vi "auto cross defense.vi"(8 "Defense type":dbl, 11 "Distance":dbl=24.0 format="%#_13g") -> ()   [LabVIEW 2015]
uses:
  <vilib>/Rock Robotics/WPI/Solenoid/WPI_SolenoidValue.ctl
  <vilib>/Rock Robotics/WPI/Solenoid/WPI_SolenoidSetEnum.vi
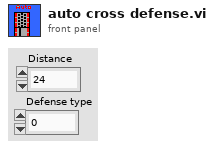
[diagram p1: front panel]
types:
  T1 = typedef "WPI_MotorControlDeviceRef.ctl" = cluster{"DeviceStatus":errorcluster, "Type":T2, "PWM":cluster{"PWM Channel":T3, "DeadBand":T4}, "CAN":cluster{"Device Number":u8, "Control Mode":T5, "Semaphore":T6, "Max Vout":dbl, "TalonSRX Control Mode":T7}, "Invert":bool}
  T2 = typedef "WPI_MotorControlType.ctl" = enum16{"PWM", "CAN", "CANTalonSRX"}
  T3 = typedef "FPGA_DIOPWMChannel.ctl" = enum8{"PWM 0", "PWM 1", "PWM 2", "PWM 3", "PWM 4", "PWM 5", "PWM 6", "PWM 7", "PWM 8", "PWM 9", "PWM MXP 0", "PWM MXP 1", "PWM MXP 2", "PWM MXP 3", "PWM MXP 4", "PWM MXP 5", "PWM MXP 6", "PWM MXP 7", "PWM MXP 8", "PWM MXP 9", "Invalid"}
  T4 = typedef "WPI_PWMDeadband.ctl" = cluster{"Name":string, "maxPositivePwm":i32, "minPositivePwm":i32, "centerPwm":i32, "maxNegativePwm":i32, "minNegativePwm":i32, "angularRange":u16}
  T5 = typedef "WPI_CANJaguar_ControlMode.ctl" = enum8{"Percent VBus", "Current", "Speed", "Position", "Voltage"}
  T6 = typedef "Semaphore RefNum" = refnum<k1>
  T7 = typedef "WPI_CANTalonSRX_APIControlMode.ctl" = enum8{"Percent VBus", "Speed", "Position", "Slave", "Unchanged / Invalid", "Voltage Compensation", "Current", "Motion Profile"}
  T8 = typedef "WPI_SolenoidDevRef.ctl" = cluster{"DevStatus":errorcluster, "Pneumatics Control Module":u8, "Forward Solenoid Channel":T9, "Reverse Solenoid Channel":T9}
  T9 = typedef "WPI_SolenoidChannel.ctl" = enum8{"Solenoid 0", "Solenoid 1", "Solenoid 2", "Solenoid 3", "Solenoid 4", "Solenoid 5", "Solenoid 6", "Solenoid 7", "Invalid"}
  T10 = typedef "WPI_SolenoidValue.ctl" = enum16{"Off", "On", "Forward", "Reverse"}
  T11 = typedef "WPI_CANTalonSRX_GlobalStatus.ctl" = cluster{"Applied Throttle":dbl, "Module Enabled":bool, "CAN Error":errorcluster, "Closed Loop Error":dbl, "Forward Limit Switch Closed":bool, "Reverse Limit Switch Closed":bool, "Sensor Position":dbl, "Sensor Velocity":dbl, "Current":dbl, "Sticky Fault - Over Temp":bool, "Sticky Fault - Under Voltage":bool, "Sticky Fault - Forward Limit":bool, "Sticky Fault - Reverse Limit":bool, "Sticky Fault - Forward Soft Limit":bool, "Sticky Fault - Reverse Soft Limit":bool, "Brake is Enabled":bool, "Encoder Position":dbl, "Encoder Velocity":dbl, "Encoder Index Count":dbl, "Encoder A Pin State":bool, "Encoder B Pin State":bool, "Encoder Index Pin State":bool, "Analog In":dbl, "Analog In Velocity":dbl, "Temperature (C)":dbl, "Battery Voltage":dbl, "Control 5 Is Supported":bool, "Current Profile Slot Select":dbl, "Pos Div 8":bool, "Vel Div 4":bool, "Pulse Width Position":i32, "Pulse Width Velocity":i32, "Pulse Width Rise To Rise (us)":i32, "Pulse Width Rise To Fall (us)":i32, "Mot Prof Active Is Under Run":bool, "Mot Prof Active Has Under Run":bool, "Mot Prof Active Is Last":bool, "Mot Prof Active Velocity Only":bool, "Mot Prof Active Is Valid":bool, "Mot Prof Buffer Is Full":bool, "Mot Prof Active Profile Slot Select":i32, "Mot Prof NextID":i32, "Mot Prof Count":i32, "Mot Prof Active Velocity":dbl, "Mot Prof Active Position":dbl, "Mot Prof Output Enable":i32}
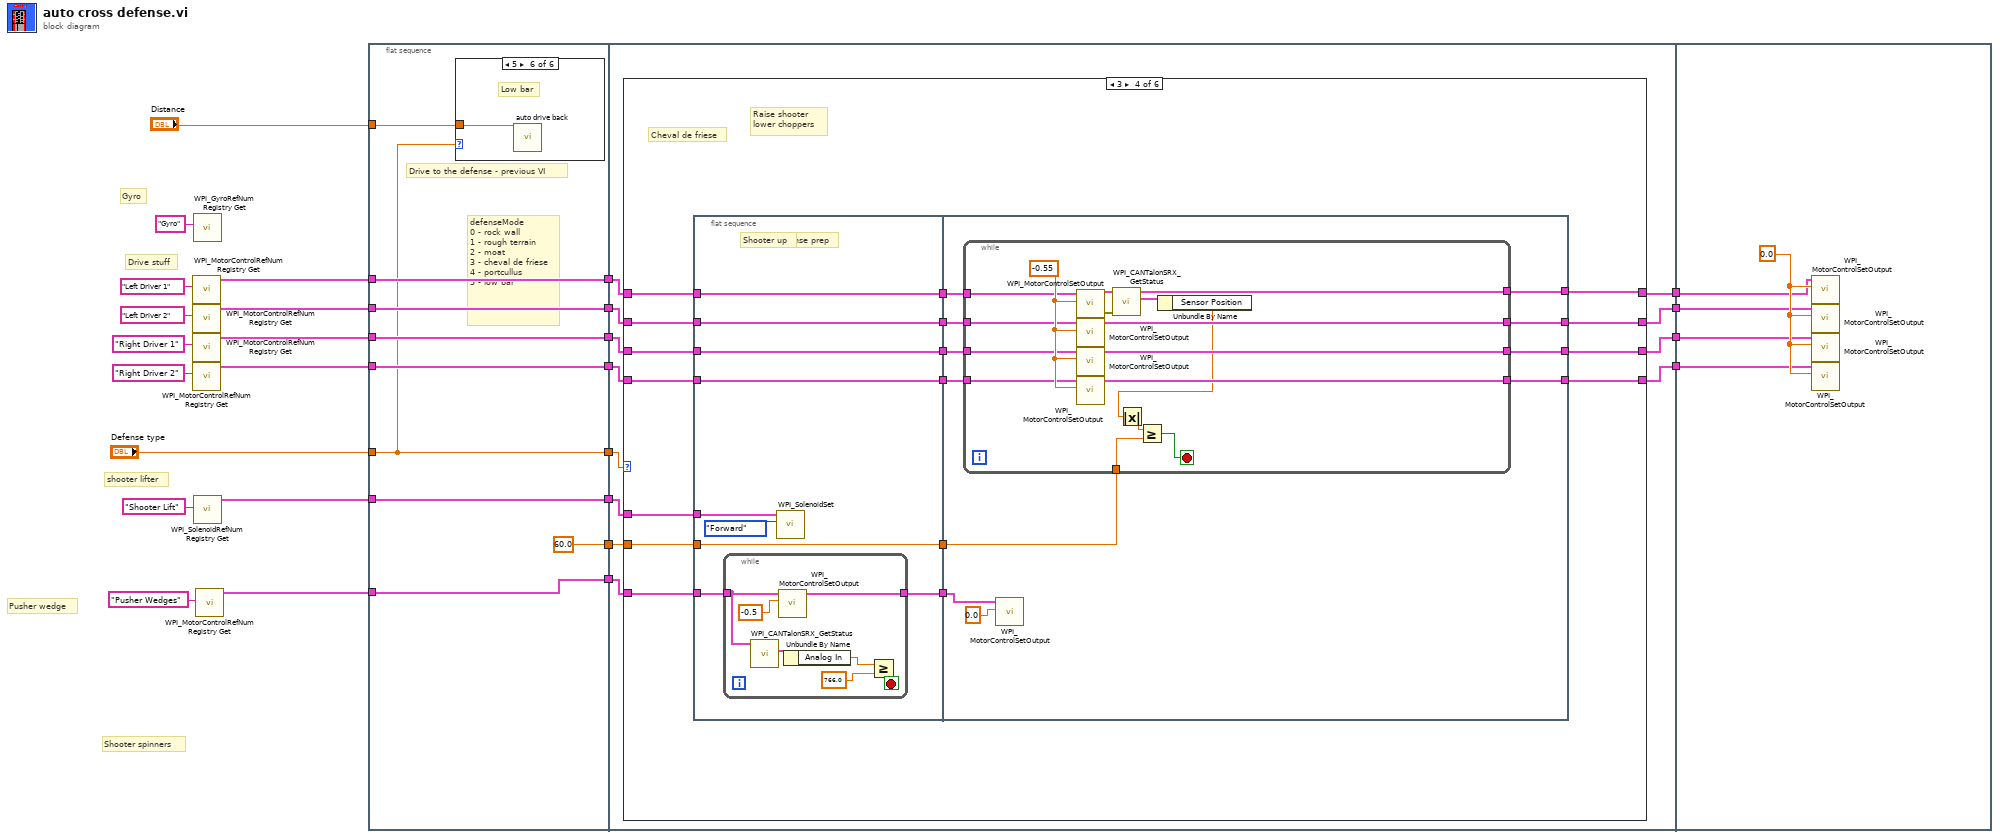
[diagram p0: block diagram]
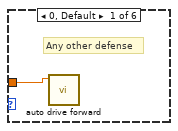
[diagram p2: hidden frame]
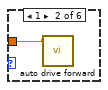
[diagram p3: hidden frame]
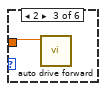
[diagram p4: hidden frame]
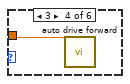
[diagram p5: hidden frame]
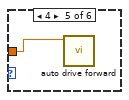
[diagram p6: hidden frame]
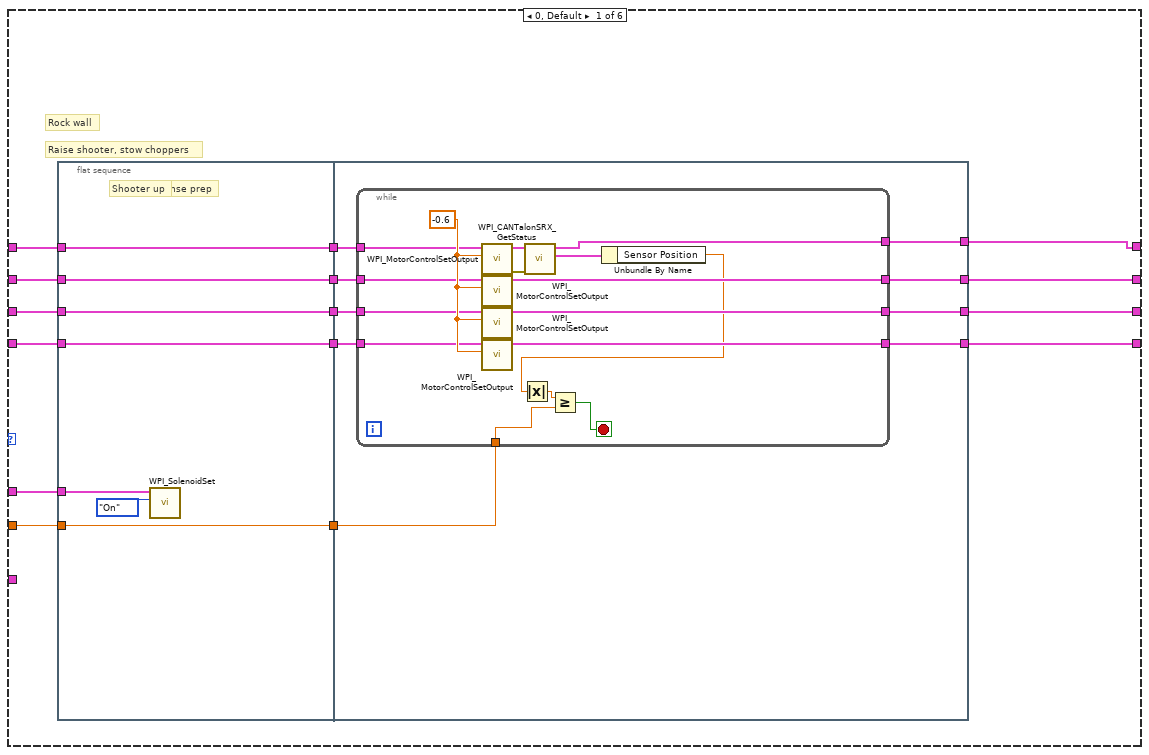
[diagram p7: hidden frame]
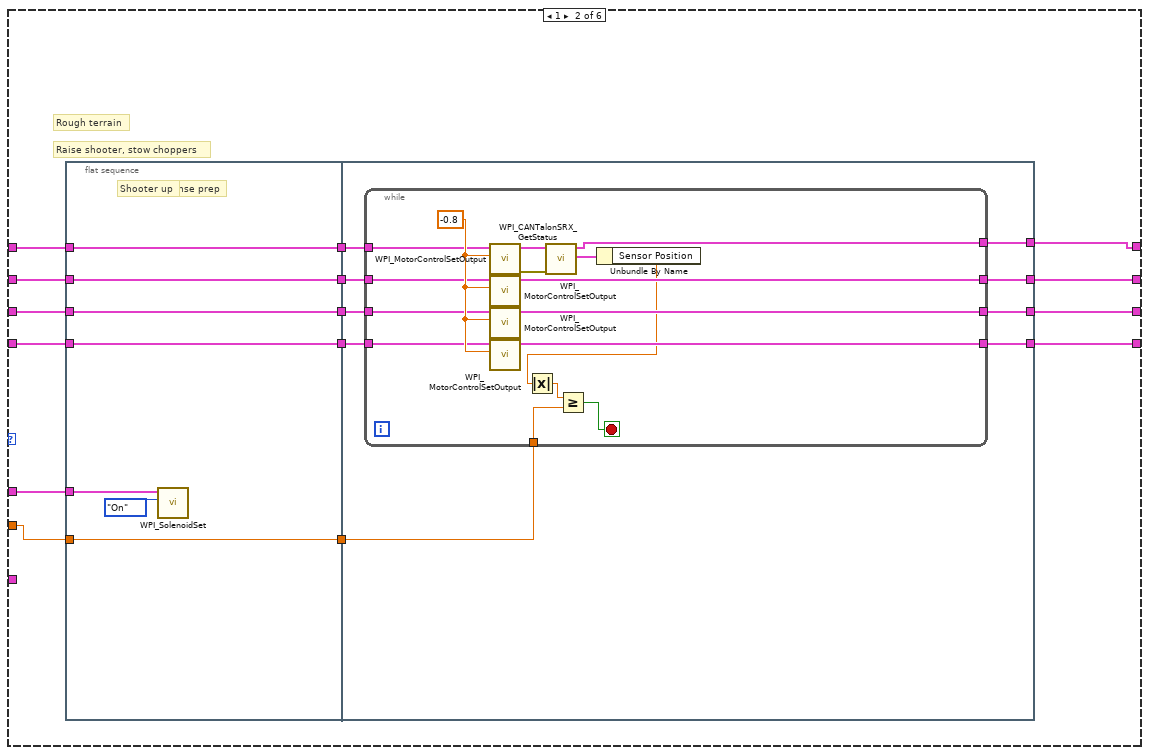
[diagram p8: hidden frame]
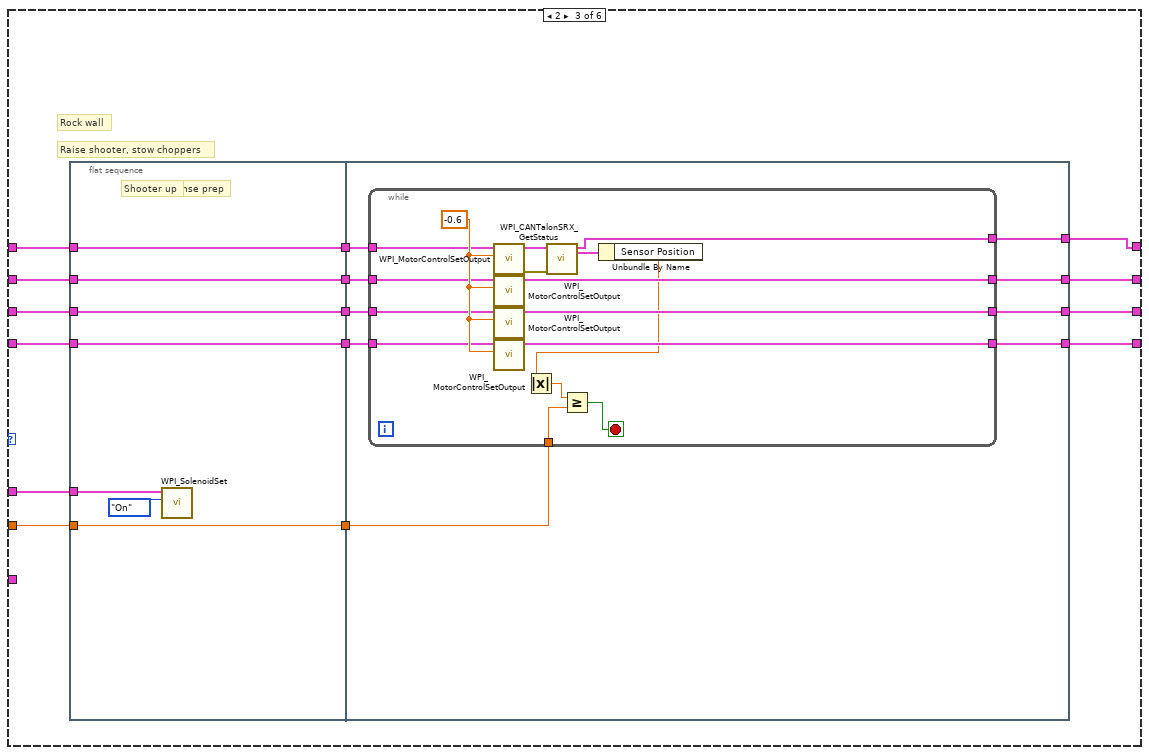
[diagram p9: hidden frame]
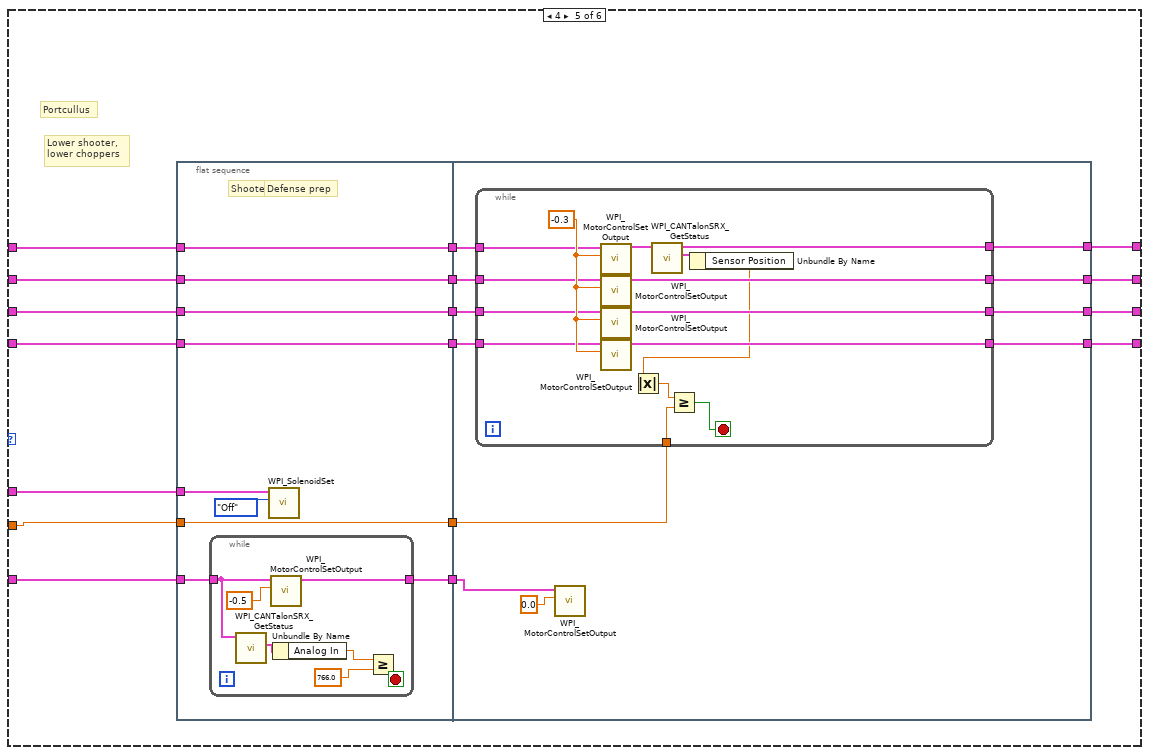
[diagram p10: hidden frame]
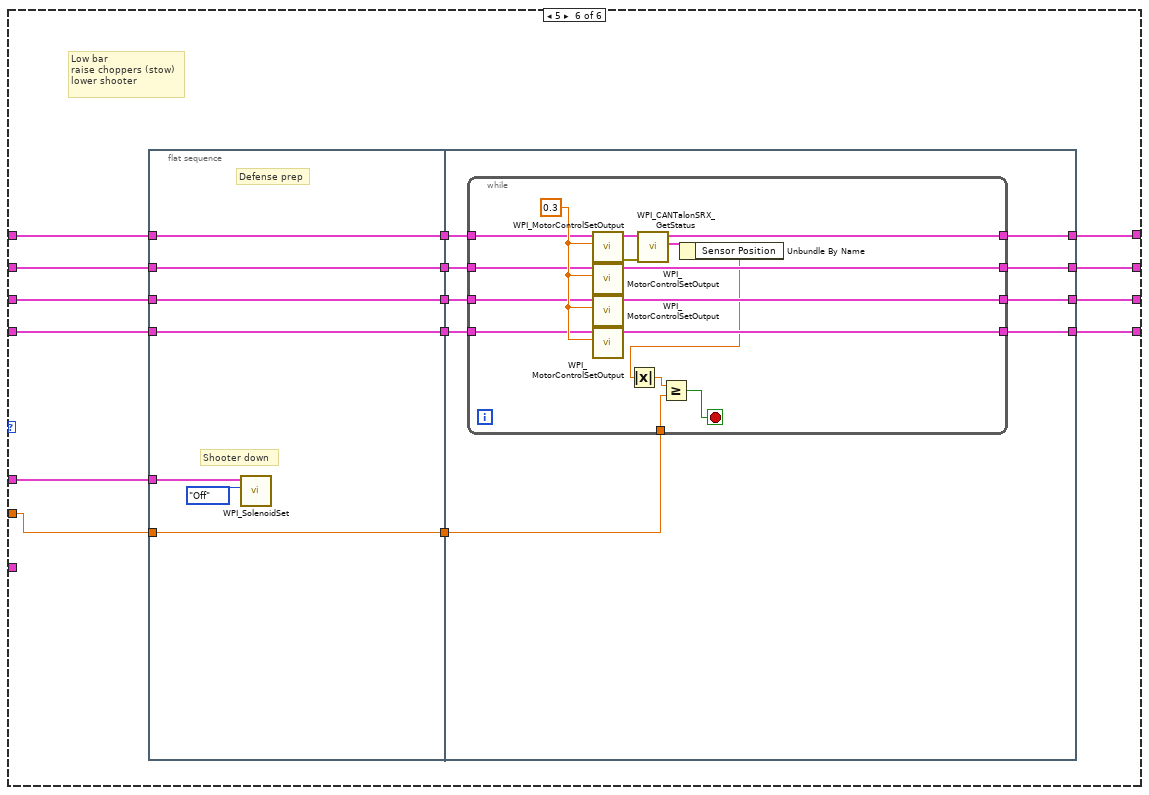
[diagram p11: hidden frame]
diagram:
  # "Pusher wedge"
  # "Shooter spinners"
  # "shooter lifter"
  # "Drive stuff"
  # "Gyro"
  n1 = call <vilib>:"WPI_MotorControlRefNum Registry Get.vi"("refnum name"="Left Driver 1") -> ("MotorControlDevRef"=w17:T1)  [unwired: 9 in, 1 out]
  n2 = call <vilib>:"WPI_MotorControlRefNum Registry Get.vi"("refnum name"="Left Driver 2") -> ("MotorControlDevRef"=w15:T1)  [unwired: 9 in, 1 out]
  n3 = call <vilib>:"WPI_MotorControlRefNum Registry Get.vi"("refnum name"="Right Driver 1") -> ("MotorControlDevRef"=w14:T1)  [unwired: 9 in, 1 out]
  n4 = call <vilib>:"WPI_MotorControlRefNum Registry Get.vi"("refnum name"="Right Driver 2") -> ("MotorControlDevRef"=w11:T1)  [unwired: 9 in, 1 out]
  n5 = call <vilib>:"WPI_GyroRefNum Registry Get.vi"("refnum name"="Gyro") -> ()  [unwired: 9 in, 2 out]
  n6 = call <vilib>:"WPI_SolenoidRefNum Registry Get.vi"("refnum name"="Shooter Lift") -> ("SolenoidDevRef"=w20:T8)  [unwired: 9 in, 1 out]
  n7 = call <vilib>:"WPI_MotorControlRefNum Registry Get.vi"("refnum name"="Pusher Wedges") -> ("MotorControlDevRef"=w3:T1)  [unwired: 9 in, 1 out]
  n8 = flat-sequence {
    tunnel: [w30] -> w21
    tunnel: "Defense type" -> [w30]
    tunnel: w20 -> [w36]
    tunnel: [w36] -> w19
    tunnel: [w35] -> w18
    tunnel: w17 -> [w35]
    tunnel: [w34] -> w16
    tunnel: w15 -> [w34]
    tunnel: w14 -> [w33]
    tunnel: [w33] -> w13
    tunnel: [w32] -> w12
    tunnel: w11 -> [w32]
    tunnel: "Distance" -> [w31]
    tunnel: [w29] -> w4
    tunnel: w3 -> [w29]
    tunnel: [60.0 ("y")] -> w2
    tunnel: w21 -> [w54]
    tunnel: w19 -> [w53]
    tunnel: w18 -> [w52]
    tunnel: w16 -> [w51]
    tunnel: w13 -> [w50]
    tunnel: w12 -> [w49]
    tunnel: [w48] -> w10
    tunnel: [w47] -> w9
    tunnel: [w46] -> w8
    tunnel: w4 -> [w45]
    tunnel: w2 -> [w44]
    tunnel: [w43] -> w1
    tunnel: w10 -> [w365]
    tunnel: w9 -> [w364]
    tunnel: w8 -> [w363]
    tunnel: w1 -> [w362]
    frame #0 {
      # "defenseMode\n0 - rock wall\n1 - rough terrain\n2 - moat\n3 - cheval de friese\n4 - portcullus\n5 - low bar"
      # "Drive to the defense - previous VI"
      n9 = case shown="5" w30 {
        tunnel: w31 -> [w37 w38 w39 w40 w41 w42]
        frame 0, Default {
          # "Any other defense"
          n10 = call "auto drive forward.vi"("Distance"=w37) -> ()  [unwired: 11 in]
        }
        frame 1 {
          n11 = call "auto drive forward.vi"("Distance"=w38) -> ()  [unwired: 11 in]
        }
        frame 2 {
          n12 = call "auto drive forward.vi"("Distance"=w39) -> ()  [unwired: 11 in]
        }
        frame 3 {
          n13 = call "auto drive forward.vi"("Distance"=w40) -> ()  [unwired: 11 in]
        }
        frame 4 {
          n14 = call "auto drive forward.vi"("Distance"=w41) -> ()  [unwired: 11 in]
        }
        frame 5 {
          # "Low bar"
          n15 = call "auto drive back.vi"("Distance"=w42) -> ()  [unwired: 11 in]
        }
      }
    }
    frame #1 {
      n16 = case shown="3" w54 {
        tunnel: w53 -> [w69 w108 w155 w203 w264 w321]
        tunnel: w52 -> [w67 w112 w159 w207 w268 w325]
        tunnel: w51 -> [w65 w111 w158 w206 w267 w324]
        tunnel: w50 -> [w64 w110 w157 w205 w266 w323]
        tunnel: w49 -> [w61 w109 w156 w204 w265 w322]
        tunnel: [w60 w107 w154 w202 w262 w318] -> w48
        tunnel: [w59 w106 w153 w201 w261 w319] -> w47
        tunnel: [w58 w105 w152 w200 w260 w320] -> w46
        tunnel: w45 -> [_ _ _ w199 w259 _]
        tunnel: w44 -> [w57 w104 w150 w198 w258 w317]
        tunnel: [w55 w102 w149 w196 w256 w315] -> w43
        frame 0, Default {
          # "Raise shooter, stow choppers"
          # "Rock wall"
          n17 = flat-sequence {
            tunnel: w69 -> [w76]
            tunnel: [w74] -> w68
            tunnel: w67 -> [w74]
            tunnel: [w73] -> w66
            tunnel: w65 -> [w73]
            tunnel: w64 -> [w72]
            tunnel: [w72] -> w63
            tunnel: [w71] -> w62
            tunnel: w61 -> [w71]
            tunnel: w57 -> [w70]
            tunnel: [w70] -> w56
            tunnel: w68 -> [w85]
            tunnel: w66 -> [w84]
            tunnel: w63 -> [w83]
            tunnel: w62 -> [w82]
            tunnel: [w81] -> w60
            tunnel: [w80] -> w59
            tunnel: [w79] -> w58
            tunnel: w56 -> [w78]
            tunnel: [w77] -> w55
            frame #0 {
              # "Defense prep"
              # "Shooter up"
              n18 = call-poly <vilib>:"WPI_SolenoidSet.vi"("Value"=WPI_SolenoidValue."On", "SolenoidDevRef"=w76) -> ()  [unwired: 8 in, 2 out]
            }
            frame #1 {
              n19 = while {
                tunnel: w85 -> [w100]
                tunnel: w84 -> [w99]
                tunnel: w83 -> [w98]
                tunnel: w82 -> [w97]
                tunnel: [w95] -> w81
                tunnel: [w94] -> w80
                tunnel: [w93] -> w79
                tunnel: w78 -> [w92]
                tunnel: [w86] -> w77
                stop <- w96 stop-if-true
                w101 = -0.6
                n20 = call <vilib>:"WPI_MotorControlSetOutput.vi"("Output"=w101, "MotorControlDevRef"=w100) -> ("error out"=w91:errorcluster, "MotorControlDevRef"=w90:T1)  [unwired: 7 in, 1 out]
                n21 = call <vilib>:"WPI_MotorControlSetOutput.vi"("Output"=w101, "MotorControlDevRef"=w99) -> ("MotorControlDevRef"=w95:T1)  [unwired: 7 in, 2 out]
                n22 = call <vilib>:"WPI_MotorControlSetOutput.vi"("Output"=w101, "MotorControlDevRef"=w98) -> ("MotorControlDevRef"=w94:T1)  [unwired: 7 in, 2 out]
                n23 = call <vilib>:"WPI_MotorControlSetOutput.vi"("Output"=w101, "MotorControlDevRef"=w97) -> ("MotorControlDevRef"=w93:T1)  [unwired: 7 in, 2 out]
                n24 = call <vilib>:"WPI_CANTalonSRX_GetStatus.vi"("error in (no error)"=w91, "CAN Talon SRX Ref"=w90) -> ("Talon SRX Status"=w89:T11, "CAN Talon SRX Ref"=w86:T1)  [unwired: 7 in, 1 out]
                n25 = Unbundle By Name(w89) -> ("Sensor Position"=w87:dbl)
                n26 = Absolute Value(x=w87) -> (abs(x)=w88:dbl)
                n27 = Greater Or Equal?(x=w88, y=w92) -> (x >= y?=w96:bool)
              }
            }
          }
        }
        frame 1 {
          # "Raise shooter, stow choppers"
          # "Rough terrain"
          n28 = flat-sequence {
            tunnel: w108 -> [w123]
            tunnel: [w121] -> w116
            tunnel: w112 -> [w121]
            tunnel: [w120] -> w115
            tunnel: w111 -> [w120]
            tunnel: w110 -> [w119]
            tunnel: [w119] -> w114
            tunnel: [w118] -> w113
            tunnel: w109 -> [w118]
            tunnel: w104 -> [w117]
            tunnel: [w117] -> w103
            tunnel: w116 -> [w132]
            tunnel: w115 -> [w131]
            tunnel: w114 -> [w130]
            tunnel: w113 -> [w129]
            tunnel: [w128] -> w107
            tunnel: [w127] -> w106
            tunnel: [w126] -> w105
            tunnel: w103 -> [w125]
            tunnel: [w124] -> w102
            frame #0 {
              # "Defense prep"
              # "Shooter up"
              n29 = call-poly <vilib>:"WPI_SolenoidSet.vi"("Value"=WPI_SolenoidValue."On", "SolenoidDevRef"=w123) -> ()  [unwired: 8 in, 2 out]
            }
            frame #1 {
              n30 = while {
                tunnel: w132 -> [w147]
                tunnel: w131 -> [w146]
                tunnel: w130 -> [w145]
                tunnel: w129 -> [w144]
                tunnel: [w142] -> w128
                tunnel: [w141] -> w127
                tunnel: [w140] -> w126
                tunnel: w125 -> [w138]
                tunnel: [w133] -> w124
                stop <- w143 stop-if-true
                w148 = -0.8
                n31 = call <vilib>:"WPI_MotorControlSetOutput.vi"("Output"=w148, "MotorControlDevRef"=w147) -> ("error out"=w137:errorcluster, "MotorControlDevRef"=w136:T1)  [unwired: 7 in, 1 out]
                n32 = call <vilib>:"WPI_MotorControlSetOutput.vi"("Output"=w148, "MotorControlDevRef"=w146) -> ("MotorControlDevRef"=w142:T1)  [unwired: 7 in, 2 out]
                n33 = call <vilib>:"WPI_MotorControlSetOutput.vi"("Output"=w148, "MotorControlDevRef"=w145) -> ("MotorControlDevRef"=w141:T1)  [unwired: 7 in, 2 out]
                n34 = call <vilib>:"WPI_MotorControlSetOutput.vi"("Output"=w148, "MotorControlDevRef"=w144) -> ("MotorControlDevRef"=w140:T1)  [unwired: 7 in, 2 out]
                n35 = call <vilib>:"WPI_CANTalonSRX_GetStatus.vi"("error in (no error)"=w137, "CAN Talon SRX Ref"=w136) -> ("Talon SRX Status"=w135:T11, "CAN Talon SRX Ref"=w133:T1)  [unwired: 7 in, 1 out]
                n36 = Unbundle By Name(w135) -> ("Sensor Position"=w134:dbl)
                n37 = Absolute Value(x=w134) -> (abs(x)=w139:dbl)
                n38 = Greater Or Equal?(x=w139, y=w138) -> (x >= y?=w143:bool)
              }
            }
          }
        }
        frame 2 {
          # "Raise shooter, stow choppers"
          # "Rock wall"
          n39 = flat-sequence {
            tunnel: w155 -> [w170]
            tunnel: [w168] -> w163
            tunnel: w159 -> [w168]
            tunnel: [w167] -> w162
            tunnel: w158 -> [w167]
            tunnel: w157 -> [w166]
            tunnel: [w166] -> w161
            tunnel: [w165] -> w160
            tunnel: w156 -> [w165]
            tunnel: [w164] -> w151
            tunnel: w150 -> [w164]
            tunnel: w163 -> [w179]
            tunnel: w162 -> [w178]
            tunnel: w161 -> [w177]
            tunnel: w160 -> [w176]
            tunnel: [w175] -> w154
            tunnel: [w174] -> w153
            tunnel: [w173] -> w152
            tunnel: w151 -> [w172]
            tunnel: [w171] -> w149
            frame #0 {
              # "Defense prep"
              # "Shooter up"
              n40 = call-poly <vilib>:"WPI_SolenoidSet.vi"("Value"=WPI_SolenoidValue."On", "SolenoidDevRef"=w170) -> ()  [unwired: 8 in, 2 out]
            }
            frame #1 {
              n41 = while {
                tunnel: w179 -> [w194]
                tunnel: w178 -> [w193]
                tunnel: w177 -> [w192]
                tunnel: w176 -> [w191]
                tunnel: [w189] -> w175
                tunnel: [w188] -> w174
                tunnel: [w187] -> w173
                tunnel: w172 -> [w185]
                tunnel: [w180] -> w171
                stop <- w190 stop-if-true
                w195 = -0.6
                n42 = call <vilib>:"WPI_MotorControlSetOutput.vi"("Output"=w195, "MotorControlDevRef"=w194) -> ("error out"=w184:errorcluster, "MotorControlDevRef"=w183:T1)  [unwired: 7 in, 1 out]
                n43 = call <vilib>:"WPI_MotorControlSetOutput.vi"("Output"=w195, "MotorControlDevRef"=w193) -> ("MotorControlDevRef"=w189:T1)  [unwired: 7 in, 2 out]
                n44 = call <vilib>:"WPI_MotorControlSetOutput.vi"("Output"=w195, "MotorControlDevRef"=w192) -> ("MotorControlDevRef"=w188:T1)  [unwired: 7 in, 2 out]
                n45 = call <vilib>:"WPI_MotorControlSetOutput.vi"("Output"=w195, "MotorControlDevRef"=w191) -> ("MotorControlDevRef"=w187:T1)  [unwired: 7 in, 2 out]
                n46 = call <vilib>:"WPI_CANTalonSRX_GetStatus.vi"("error in (no error)"=w184, "CAN Talon SRX Ref"=w183) -> ("Talon SRX Status"=w182:T11, "CAN Talon SRX Ref"=w180:T1)  [unwired: 7 in, 1 out]
                n47 = Unbundle By Name(w182) -> ("Sensor Position"=w181:dbl)
                n48 = Absolute Value(x=w181) -> (abs(x)=w186:dbl)
                n49 = Greater Or Equal?(x=w186, y=w185) -> (x >= y?=w190:bool)
              }
            }
          }
        }
        frame 3 {
          # "Raise shooter\nlower choppers"
          # "Cheval de friese"
          n50 = flat-sequence {
            tunnel: w203 -> [w221]
            tunnel: [w219] -> w212
            tunnel: w207 -> [w219]
            tunnel: [w218] -> w211
            tunnel: w206 -> [w218]
            tunnel: w205 -> [w217]
            tunnel: [w217] -> w210
            tunnel: [w216] -> w209
            tunnel: w204 -> [w216]
            tunnel: [w215] -> w208
            tunnel: w199 -> [w214]
            tunnel: w198 -> [w213]
            tunnel: [w213] -> w197
            tunnel: w212 -> [w239]
            tunnel: w211 -> [w238]
            tunnel: w210 -> [w237]
            tunnel: w209 -> [w236]
            tunnel: w208 -> [w231]
            tunnel: w197 -> [w230]
            tunnel: [w235] -> w202
            tunnel: [w234] -> w201
            tunnel: [w233] -> w200
            tunnel: [w229] -> w196
            frame #0 {
              # "Defense prep"
              # "Shooter up"
              n51 = while {
                tunnel: [w227] -> w215
                tunnel: w214 -> [w222]
                stop <- w223 stop-if-true
                n52 = call <vilib>:"WPI_CANTalonSRX_GetStatus.vi"("CAN Talon SRX Ref"=w222) -> ("Talon SRX Status"=w225:T11)  [unwired: 8 in, 2 out]
                n53 = call <vilib>:"WPI_MotorControlSetOutput.vi"("Output"=-0.5, "MotorControlDevRef"=w222) -> ("MotorControlDevRef"=w227:T1)  [unwired: 7 in, 2 out]
                n54 = Unbundle By Name(w225) -> ("Analog In"=w224:dbl)
                n55 = Greater Or Equal?(x=w224, y=766.0) -> (x >= y?=w223:bool)
              }
              n56 = call-poly <vilib>:"WPI_SolenoidSet.vi"("Value"=WPI_SolenoidValue."Forward", "SolenoidDevRef"=w221) -> ()  [unwired: 8 in, 2 out]
            }
            frame #1 {
              n57 = while {
                tunnel: w239 -> [w254]
                tunnel: w238 -> [w253]
                tunnel: w237 -> [w252]
                tunnel: w236 -> [w251]
                tunnel: [w249] -> w235
                tunnel: [w248] -> w234
                tunnel: [w247] -> w233
                tunnel: w230 -> [w245]
                tunnel: [w240] -> w229
                stop <- w250 stop-if-true
                w255 = -0.55
                n58 = call <vilib>:"WPI_MotorControlSetOutput.vi"("Output"=w255, "MotorControlDevRef"=w254) -> ("error out"=w243:errorcluster, "MotorControlDevRef"=w244:T1)  [unwired: 7 in, 1 out]
                n59 = call <vilib>:"WPI_MotorControlSetOutput.vi"("Output"=w255, "MotorControlDevRef"=w253) -> ("MotorControlDevRef"=w249:T1)  [unwired: 7 in, 2 out]
                n60 = call <vilib>:"WPI_MotorControlSetOutput.vi"("Output"=w255, "MotorControlDevRef"=w252) -> ("MotorControlDevRef"=w248:T1)  [unwired: 7 in, 2 out]
                n61 = call <vilib>:"WPI_MotorControlSetOutput.vi"("Output"=w255, "MotorControlDevRef"=w251) -> ("MotorControlDevRef"=w247:T1)  [unwired: 7 in, 2 out]
                n62 = call <vilib>:"WPI_CANTalonSRX_GetStatus.vi"("error in (no error)"=w243, "CAN Talon SRX Ref"=w244) -> ("Talon SRX Status"=w242:T11, "CAN Talon SRX Ref"=w240:T1)  [unwired: 7 in, 1 out]
                n63 = Unbundle By Name(w242) -> ("Sensor Position"=w241:dbl)
                n64 = Absolute Value(x=w241) -> (abs(x)=w246:dbl)
                n65 = Greater Or Equal?(x=w246, y=w245) -> (x >= y?=w250:bool)
              }
              n66 = call <vilib>:"WPI_MotorControlSetOutput.vi"("Output"=0.0, "MotorControlDevRef"=w231) -> ()  [unwired: 7 in, 3 out]
            }
          }
        }
        frame 4 {
          # "Lower shooter,\nlower choppers"
          # "Portcullus"
          n67 = flat-sequence {
            tunnel: w264 -> [w281]
            tunnel: [w279] -> w272
            tunnel: w268 -> [w279]
            tunnel: [w278] -> w271
            tunnel: w267 -> [w278]
            tunnel: w266 -> [w277]
            tunnel: [w277] -> w270
            tunnel: [w276] -> w269
            tunnel: w265 -> [w276]
            tunnel: [w275] -> w263
            tunnel: w259 -> [w274]
            tunnel: w258 -> [w273]
            tunnel: [w273] -> w257
            tunnel: w272 -> [w299]
            tunnel: w271 -> [w298]
            tunnel: w270 -> [w297]
            tunnel: w269 -> [w296]
            tunnel: w263 -> [w291]
            tunnel: w257 -> [w290]
            tunnel: [w295] -> w262
            tunnel: [w294] -> w261
            tunnel: [w293] -> w260
            tunnel: [w289] -> w256
            frame #0 {
              # "Defense prep"
              # "Shooter down"
              n68 = while {
                tunnel: [w287] -> w275
                tunnel: w274 -> [w282]
                stop <- w283 stop-if-true
                n69 = call <vilib>:"WPI_CANTalonSRX_GetStatus.vi"("CAN Talon SRX Ref"=w282) -> ("Talon SRX Status"=w285:T11)  [unwired: 8 in, 2 out]
                n70 = call <vilib>:"WPI_MotorControlSetOutput.vi"("Output"=-0.5, "MotorControlDevRef"=w282) -> ("MotorControlDevRef"=w287:T1)  [unwired: 7 in, 2 out]
                n71 = Unbundle By Name(w285) -> ("Analog In"=w284:dbl)
                n72 = Greater Or Equal?(x=w284, y=766.0) -> (x >= y?=w283:bool)
              }
              n73 = call-poly <vilib>:"WPI_SolenoidSet.vi"("Value"=WPI_SolenoidValue."Off", "SolenoidDevRef"=w281) -> ()  [unwired: 8 in, 2 out]
            }
            frame #1 {
              n74 = while {
                tunnel: w299 -> [w313]
                tunnel: w298 -> [w312]
                tunnel: w297 -> [w311]
                tunnel: w296 -> [w310]
                tunnel: [w308] -> w295
                tunnel: [w307] -> w294
                tunnel: [w306] -> w293
                tunnel: w290 -> [w304]
                tunnel: [w302] -> w289
                stop <- w309 stop-if-true
                w314 = -0.3
                n75 = call <vilib>:"WPI_MotorControlSetOutput.vi"("Output"=w314, "MotorControlDevRef"=w313) -> ("MotorControlDevRef"=w303:T1)  [unwired: 7 in, 2 out]
                n76 = call <vilib>:"WPI_MotorControlSetOutput.vi"("Output"=w314, "MotorControlDevRef"=w312) -> ("MotorControlDevRef"=w308:T1)  [unwired: 7 in, 2 out]
                n77 = call <vilib>:"WPI_MotorControlSetOutput.vi"("Output"=w314, "MotorControlDevRef"=w311) -> ("MotorControlDevRef"=w307:T1)  [unwired: 7 in, 2 out]
                n78 = call <vilib>:"WPI_MotorControlSetOutput.vi"("Output"=w314, "MotorControlDevRef"=w310) -> ("MotorControlDevRef"=w306:T1)  [unwired: 7 in, 2 out]
                n79 = call <vilib>:"WPI_CANTalonSRX_GetStatus.vi"("CAN Talon SRX Ref"=w303) -> ("Talon SRX Status"=w301:T11, "CAN Talon SRX Ref"=w302:T1)  [unwired: 8 in, 1 out]
                n80 = Unbundle By Name(w301) -> ("Sensor Position"=w300:dbl)
                n81 = Absolute Value(x=w300) -> (abs(x)=w305:dbl)
                n82 = Greater Or Equal?(x=w305, y=w304) -> (x >= y?=w309:bool)
              }
              n83 = call <vilib>:"WPI_MotorControlSetOutput.vi"("Output"=0.0, "MotorControlDevRef"=w291) -> ()  [unwired: 7 in, 3 out]
            }
          }
        }
        frame 5 {
          # "Low bar\nraise choppers (stow)\nlower shooter"
          n84 = flat-sequence {
            tunnel: w321 -> [w336]
            tunnel: [w334] -> w329
            tunnel: w325 -> [w334]
            tunnel: [w333] -> w328
            tunnel: w324 -> [w333]
            tunnel: w323 -> [w332]
            tunnel: [w332] -> w327
            tunnel: [w331] -> w326
            tunnel: w322 -> [w331]
            tunnel: w317 -> [w330]
            tunnel: [w330] -> w316
            tunnel: w329 -> [w345]
            tunnel: w328 -> [w344]
            tunnel: w327 -> [w343]
            tunnel: w326 -> [w342]
            tunnel: [w341] -> w318
            tunnel: [w340] -> w319
            tunnel: [w339] -> w320
            tunnel: w316 -> [w338]
            tunnel: [w337] -> w315
            frame #0 {
              # "Defense prep"
              # "Shooter down"
              n85 = call-poly <vilib>:"WPI_SolenoidSet.vi"("Value"=WPI_SolenoidValue."Off", "SolenoidDevRef"=w336) -> ()  [unwired: 8 in, 2 out]
            }
            frame #1 {
              n86 = while {
                tunnel: w345 -> [w360]
                tunnel: w344 -> [w359]
                tunnel: w343 -> [w358]
                tunnel: w342 -> [w357]
                tunnel: [w355] -> w341
                tunnel: [w354] -> w340
                tunnel: [w353] -> w339
                tunnel: w338 -> [w351]
                tunnel: [w348] -> w337
                stop <- w356 stop-if-true
                w361 = 0.3
                n87 = call <vilib>:"WPI_MotorControlSetOutput.vi"("Output"=w361, "MotorControlDevRef"=w360) -> ("error out"=w350:errorcluster, "MotorControlDevRef"=w349:T1)  [unwired: 7 in, 1 out]
                n88 = call <vilib>:"WPI_MotorControlSetOutput.vi"("Output"=w361, "MotorControlDevRef"=w359) -> ("MotorControlDevRef"=w355:T1)  [unwired: 7 in, 2 out]
                n89 = call <vilib>:"WPI_MotorControlSetOutput.vi"("Output"=w361, "MotorControlDevRef"=w358) -> ("MotorControlDevRef"=w354:T1)  [unwired: 7 in, 2 out]
                n90 = call <vilib>:"WPI_MotorControlSetOutput.vi"("Output"=w361, "MotorControlDevRef"=w357) -> ("MotorControlDevRef"=w353:T1)  [unwired: 7 in, 2 out]
                n91 = call <vilib>:"WPI_CANTalonSRX_GetStatus.vi"("error in (no error)"=w350, "CAN Talon SRX Ref"=w349) -> ("Talon SRX Status"=w347:T11, "CAN Talon SRX Ref"=w348:T1)  [unwired: 7 in, 1 out]
                n92 = Unbundle By Name(w347) -> ("Sensor Position"=w346:dbl)
                n93 = Absolute Value(x=w346) -> (abs(x)=w352:dbl)
                n94 = Greater Or Equal?(x=w352, y=w351) -> (x >= y?=w356:bool)
              }
            }
          }
        }
      }
    }
    frame #2 {
      w366 = 0.0
      n95 = call <vilib>:"WPI_MotorControlSetOutput.vi"("Output"=w366, "MotorControlDevRef"=w362) -> ()  [unwired: 7 in, 3 out]
      n96 = call <vilib>:"WPI_MotorControlSetOutput.vi"("Output"=w366, "MotorControlDevRef"=w365) -> ()  [unwired: 7 in, 3 out]
      n97 = call <vilib>:"WPI_MotorControlSetOutput.vi"("Output"=w366, "MotorControlDevRef"=w364) -> ()  [unwired: 7 in, 3 out]
      n98 = call <vilib>:"WPI_MotorControlSetOutput.vi"("Output"=w366, "MotorControlDevRef"=w363) -> ()  [unwired: 7 in, 3 out]
    }
  }
